vi "CoboltLaser_SerialNumberGet.vi"(0 "ComPort":refnum<visa-resource-name>, 3 "GenerateError":bool=TRUE, 7 "error in (no error)":errorcluster) -> (20 "ComPortOut":refnum<visa-resource-name>, 21 "SerialNumber":string, 23 "Serial number":dbl=nan, 27 "error out":errorcluster)   [LabVIEW 2019]
doc: "Use this template to build a VI to use as a subVI."
uses:
  <userlib>/CoboltLaser/CoboltLaser_Controls/ExpectedResponseType.ctl
panel:
  out "ResponseOK":bool
  out "Response":string
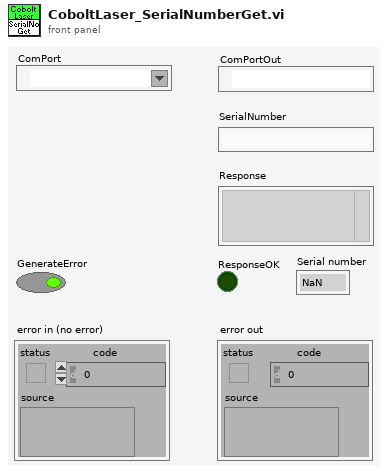
[diagram p1: front panel]
types:
  T1 = typedef "ExpectedResponseType.ctl" = enum16{"Any", "Digits Only", "Non-Digits Only"}
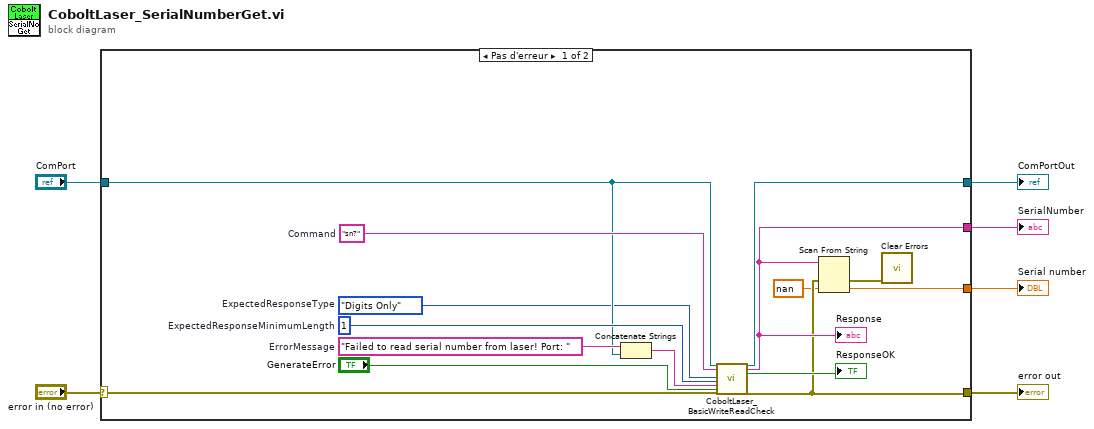
[diagram p0: block diagram]
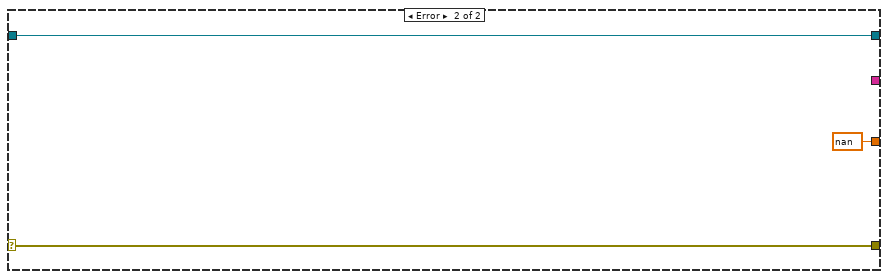
[diagram p2: hidden frame]
diagram:
  n1 = case shown="Pas d'erreur" "error in (no error)" {
    selector: "error in (no error)" -> [w21 w24]
    tunnel: [w10 w24] -> w5
    tunnel: "ComPort" -> [w14 w23]
    tunnel: [w13 w23] -> w3
    tunnel: [w12 nan] -> w2
    tunnel: [w11 _] -> w1
    frame No Error {
      w7 = ExpectedResponseType."Digits Only"  # ExpectedResponseType
      w19 = 1  # ExpectedResponseMinimumLength
      w16 = "Failed to read serial number from laser! Port: "  # ErrorMessage
      w20 = "sn?"  # Command
      n2 = Concatenate Strings(w16, w14) -> (w15:string)
      n3 = call <userlib>:"CoboltLaser_BasicWriteReadCheck.vi"("ComPort"=w14, "Command"=w20, "ExpectedResponseType"=w7, "ExpectedResponseMinimumLength"=w19, "ErrorMessage"=w15, "GenerateError"="GenerateError", "error in (no error)"=w21) -> ("ComPortOut"=w13:refnum<visa-resource-name>, "Response"=w11:string, "ResponseOK"=→"ResponseOK":bool, "error out"=w10:errorcluster)  [unwired: 17 in]
      "Response" <- w11
      n4 = Scan From String(input string=w11, error in=w10, default 1=nan ("default value 1")) -> (error out=w8:errorcluster, output 1=w12:dbl)  [unwired: 2 in, 2 out]
      n5 = call <vilib>:"Clear Errors.vi"("error in (no error)"=w8) -> ()  [unwired: 5 in, 2 out]
    }
    frame Error {
    }
  }
  "error out" <- w5
  "ComPortOut" <- w3
  "Serial number" <- w2
  "SerialNumber" <- w1
